vi "LiftRefSelector.vi"(10 "LiftRefs":T1) -> (2 "String":string)   [LabVIEW 2014, in "LiftLib.lvlib"]
uses:
  LiftLib.lvlib
  LiftRefs.ctl
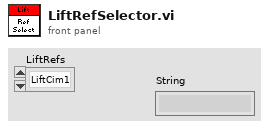
[diagram p1: front panel]
types:
  T1 = typedef "LiftLib.lvlib/LiftRefs.ctl" = enum16{"LiftCim1", "LiftCim2", "LiftEncoder", "LiftLimitSwitch1", "LiftLimitSwitch2"}
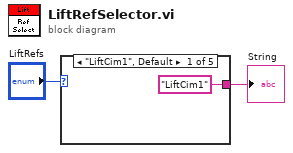
[diagram p0: block diagram]
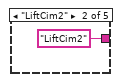
[diagram p2: hidden frame]
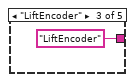
[diagram p3: hidden frame]
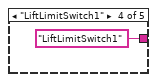
[diagram p4: hidden frame]
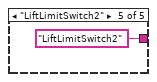
[diagram p5: hidden frame]
diagram:
  n1 = case shown="\"LiftCim1\", Default" "LiftRefs" {
    tunnel: ["LiftCim1" "LiftCim2" "LiftEncoder" "LiftLimitSwitch1" "LiftLimitSwitch2"] -> w1
    frame "LiftCim1", Default {
    }
    frame "LiftCim2" {
    }
    frame "LiftEncoder" {
    }
    frame "LiftLimitSwitch1" {
    }
    frame "LiftLimitSwitch2" {
    }
  }
  "String" <- w1
